vi "ReverseDirection.vi"(0 "reference":refnum<class "ClassRelationshipEdge.lvclass">, 5 "error in (no error)":errorcluster) -> (14 "reference out":refnum<class "ClassRelationshipEdge.lvclass">, 19 "error out":errorcluster)   [LabVIEW 2016, in "ClassRelationshipEdge.lvclass"]
uses:
  <resource>/Framework/Providers/Open_GDS/UML/ClassRelationshipEdge_class/ClassRelationshipEdge.lvclass
  <resource>/Framework/Providers/Open_GDS/UML/SegmentedLineEdge_class/SegmentedLineEdge.lvclass
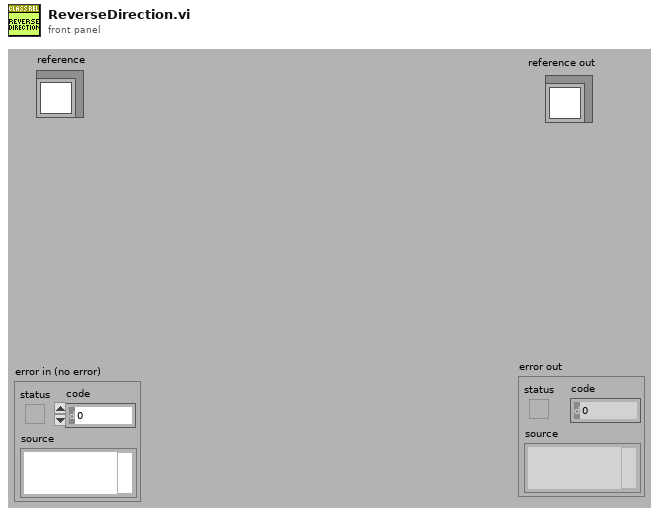
[diagram p1: front panel]
types:
  T1 = typedef "ClassRelationshipEdge.lvclass/ObjectAttributes.ctl" = cluster{"bentStyleRef":refnum<class "BentStyle.lvclass">, "startConnectionOffset":cluster{"x":i32, "y":i32}, "endConnectionOffset":cluster{"x":i32, "y":i32}, "MidLineOffset":cluster{"x":i32, "y":i32}, "DepClass":T2}
  T2 = typedef "ReversedEngineering_ViDependencyDetailsType.ctl" = cluster{"ThisVIs/Ctls":path[], "Dependent_VIs/Ctls":path[]}
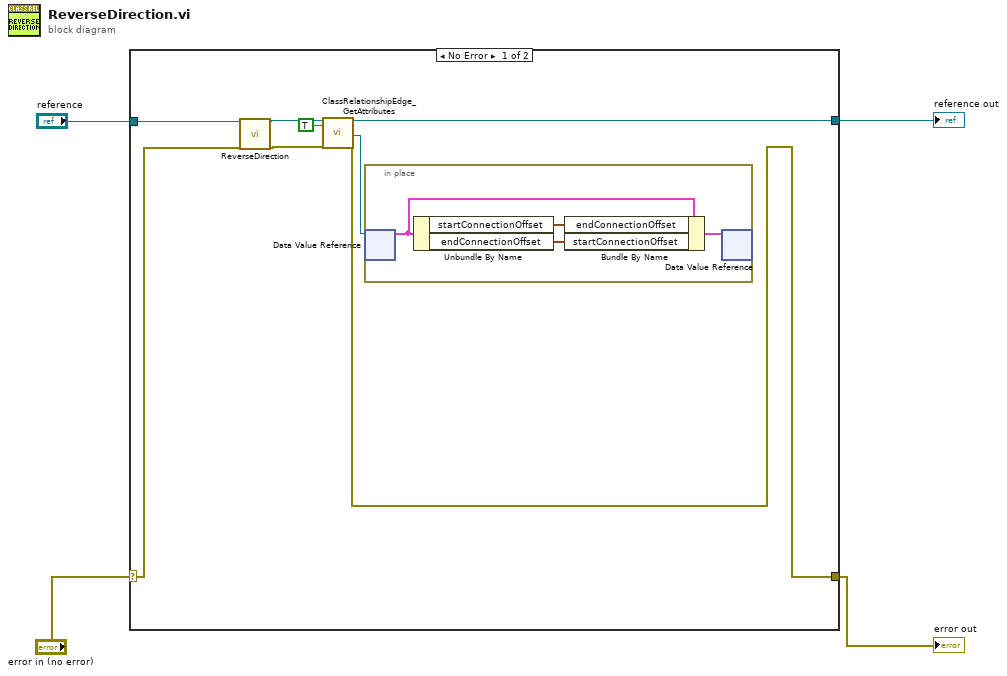
[diagram p0: block diagram]
diagram:
  n1 = case shown="No Error" "error in (no error)" {
    selector: "error in (no error)" -> [w9 w17]
    tunnel: "reference" -> [w7 w18]
    tunnel: [w12 w17] -> w2
    tunnel: [w11 w18] -> w1
    frame No Error {
      n2 = call-parent "ReverseDirection.vi"("reference"=w7, "error in (no error)"=w9) -> ("reference out"=w8:refnum<class "ClassRelationshipEdge.lvclass">, "error out"=w10:errorcluster)  [unwired: 16 in]
      n3 = call <resource>:"ClassRelationshipEdge_GetAttributes.vi"("reference in"=w8, "OnlyGetDvrReference(False)"=TRUE, "error in (no error)"=w10) -> ("reference out"=w11:refnum<class "ClassRelationshipEdge.lvclass">, "DataRef"=w5:refnum<data-value>, "error out"=w12:errorcluster)  [unwired: 13 in, 1 out]
      n4 = in-place {
        n5 = in-place-dvr #1(w5) -> (w16:T1)  [unwired: 1 out]
        n6 = Unbundle By Name(w16) -> ("startConnectionOffset"=w15:cluster{"x":i32, "y":i32}, "endConnectionOffset"=w14:cluster{"x":i32, "y":i32})
        n7 = Bundle By Name(cluster=w16, "endConnectionOffset"=w15, "startConnectionOffset"=w14) -> (w13:T1)
        n8 = in-place-dvr #1(w13) -> ()  [unwired: 2 out]
      }
    }
    frame Error {
    }
  }
  "reference out" <- w1
  "error out" <- w2
